vi "Analogue 2 (Color, Attenuator).vi"(11 "Laser Color":u32(knob) scale=0.0..3.0) -> (0 "att 7":fxp<+/-,20,5> format="%.2g", 1 "att 6":fxp<+/-,20,5> format="%.2g", 2 "att 5":fxp<+/-,20,5> format="%.2g", 3 "att 4":fxp<+/-,20,5> format="%.2g", 5 "att 3":fxp<+/-,20,5> format="%.2g", 8 "att 2":fxp<+/-,20,5> format="%.2g", 9 "att 1":fxp<+/-,20,5> format="%.2g")   [LabVIEW 2023]
uses:
  <vilib>/rvi/eio/common/nirviEmuTemplateMethod_errors.vi
  <vilib>/eio/EIONode/EIONode.xnode
panel:
  # "Analogue 2: Attenuator, Color"
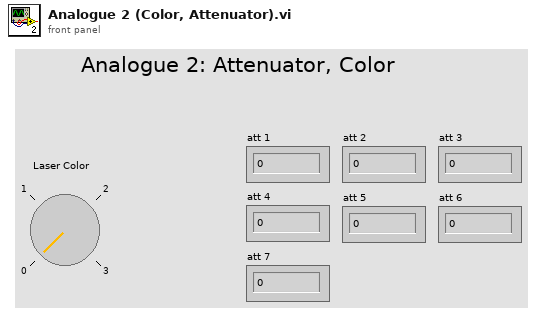
[diagram p1: front panel]
types:
  T1 = cluster{"att 1":fxp<+/-,20,5>, "att 2":fxp<+/-,20,5>, "att 3":fxp<+/-,20,5>, "att 4":fxp<+/-,20,5>, "att 5":fxp<+/-,20,5>, "att 6":fxp<+/-,20,5>, "att 7":fxp<+/-,20,5>}[]
  T2 = cluster{"att 1":fxp<+/-,20,5>, "att 2":fxp<+/-,20,5>, "att 3":fxp<+/-,20,5>, "att 4":fxp<+/-,20,5>, "att 5":fxp<+/-,20,5>, "att 6":fxp<+/-,20,5>, "att 7":fxp<+/-,20,5>}
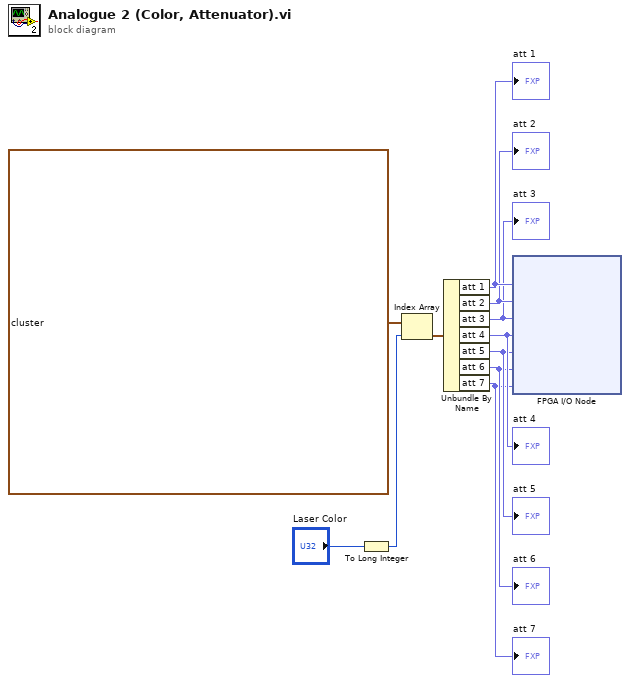
[diagram p0: block diagram]
diagram:
  n1 = To Long Integer(number="Laser Color") -> (32bit integer=w10:i32)
  n2 = Index Array(array=T1 [{"att 1"=0.0, "att 2"=0.0, "att 3"=0.0, "att 4"=0.0, "att 5"=0.0, "att 6"=0.0, "att 7"=0.0}, {"att 1"=0.0, "att 2"=0.0, "att 3"=0.0, "att 4"=0.0, "att 5"=0.0, "att 6"=0.0, "att 7"=0.0}, {"att 1"=0.0, "att 2"=0.0, "att 3"=0.0, "att 4"=0.0, "att 5"=0.0, "att 6"=0.0, "att 7"=0.0}, {"att 1"=0.0, "att 2"=0.0, "att 3"=0.0, "att 4"=0.0, "att 5"=0.0, "att 6"=0.0, "att 7"=0.0}], index=w10) -> (element=w8:T2)
  n3 = Unbundle By Name(w8) -> ("att 1"=w7:fxp<+/-,20,5>, "att 2"=w6:fxp<+/-,20,5>, "att 3"=w5:fxp<+/-,20,5>, "att 4"=w4:fxp<+/-,20,5>, "att 5"=w3:fxp<+/-,20,5>, "att 6"=w2:fxp<+/-,20,5>, "att 7"=w1:fxp<+/-,20,5>)
  "att 1" <- w7
  "att 2" <- w6
  "att 3" <- w5
  "att 4" <- w4
  "att 5" <- w3
  "att 6" <- w2
  "att 7" <- w1
  n4 = xnode "FPGA I/O Node"("Mod3/AO6"=w7, "Mod3/AO7"=w6, "Mod3/AO8"=w5, "Mod3/AO9"=w4, "Mod3/AO10"=w3, "Mod3/AO11"=w2, "Mod3/AO12"=w1) -> ()  [unwired: 7 in, 7 out]
